vi "下移动.vi"(3 "移动前":u16[][](array[numeric])=[[0, 0, 6, 1], [0, 0, 2, 0], [0, 0, 0, 0], [0, 0, 0, 1]]) -> (0 "移动后":i32[][](array[numeric]), 1 "分数":ext)   [LabVIEW 2013]
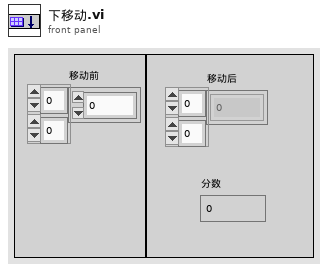
[diagram p1: front panel]
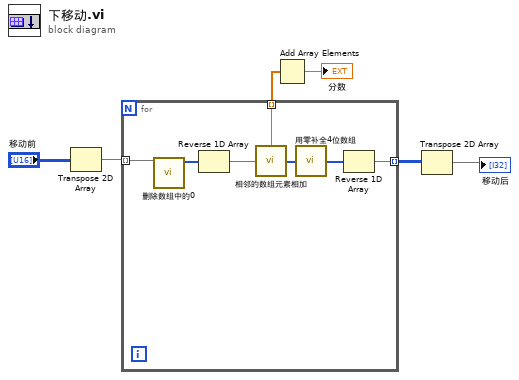
[diagram p0: block diagram]
diagram:
  n1 = Transpose 2D Array(2D array="移动前") -> (transposed array=w3:u16[][])
  n2 = for {
    tunnel: w3 -> [w13] mode=indexing
    tunnel: [w9] -> w6 mode=indexing
    tunnel: [w7] -> w2 mode=indexing
    n3 = call "删除数组中的0.vi"("数组输入"=w13) -> ("数组输出"=w11:u16[])  [unwired: 10 in]
    n4 = Reverse 1D Array(array=w11) -> (reversed array=w10:u16[])
    n5 = call "相邻的数组元素相加.vi"("数组输入"=w10) -> ("数组输出"=w12:i32[], "分数"=w7:ext)  [unwired: 2 in]
    n6 = call "用零补全4位数组.vi"("数组输入"=w12) -> ("数组输出"=w8:i32[])
    n7 = Reverse 1D Array(array=w8) -> (reversed array=w9:i32[])
  }
  n8 = Add Array Elements(numeric array=w2) -> (sum=→"分数":ext)
  n9 = Transpose 2D Array(2D array=w6) -> (transposed array=→"移动后":i32[][])
